vi "DrawFormattedMultilineString_SubVI.vi"(0 "PictureIn":picture, 1 "FormattedMultiLineStringIn":string="123<B>ABCD</B>456\nAAA<B>BBB<I>CCC<U>DDD</U>EEE</I>FFF</B>GGG\n<I>QWERTY</I>\n<U>D<B>123</B>D</U>E", 2 "TextRectangle":T2={"x"=10.0, "y"=10.0, "width"=150.0, "height"=200.0} {"height" format="%.2f"; "width" format="%.2f"; "y" format="%.2f"; "x" format="%.2f"}, 3 "Justification":T1=enum."RIGHT", 4 "GAP":i32, 5 "Font":T3={"Font Name:"="Arial", "Size"=14, "Strikeout?"=FALSE, "Italic?"=FALSE, "Underline?"=FALSE, "Outline?"=FALSE, "Shadow?"=FALSE, "Bold?"=FALSE}, 6 "scaleY":dbl=2.0, 7 "Color":u32(colorbox), 8 "scaleX":dbl=2.0) -> (14 "PictureOut":picture, 16 "NoChange":bool=TRUE)   [LabVIEW 2014, in "Graphics.lvclass"]
uses:
  <resource>/Framework/Providers/Open_GDS/UML/Graphics_class/Graphics.lvclass
  <resource>/Framework/Providers/Open_GDS/UML/General/Rectangle/Rectangle Rectangle2D.ctl
  <resource>/Framework/Providers/Open_GDS/UML/MultiLineString_class/JustificationType.ctl
  <resource>/Framework/Providers/Open_GDS/UML/MultiLineString_class/MultiLineString.lvclass
panel:
  # "Layout:\nRemove \\r\\n\nSplit in lines-array\nCalc width per char\nGet number of chars to use for line,\nif rest characters, add these to beggining of  lines-array.\nCalc Bound\nAdd \\r\\n where new lines breaks are"
  # "Drawing:\nRemove \\r, split line using \\n\nfor every line calc total length.\n\nFor each line\n  If left start\n  X=B.X+Gap\n  Right:\n  X=B.X+B.W-L.length-Gap\n  Center:\n  X=B.X+(B.W/2)-(L.length/2)\n  Draw Line\nEnd For"
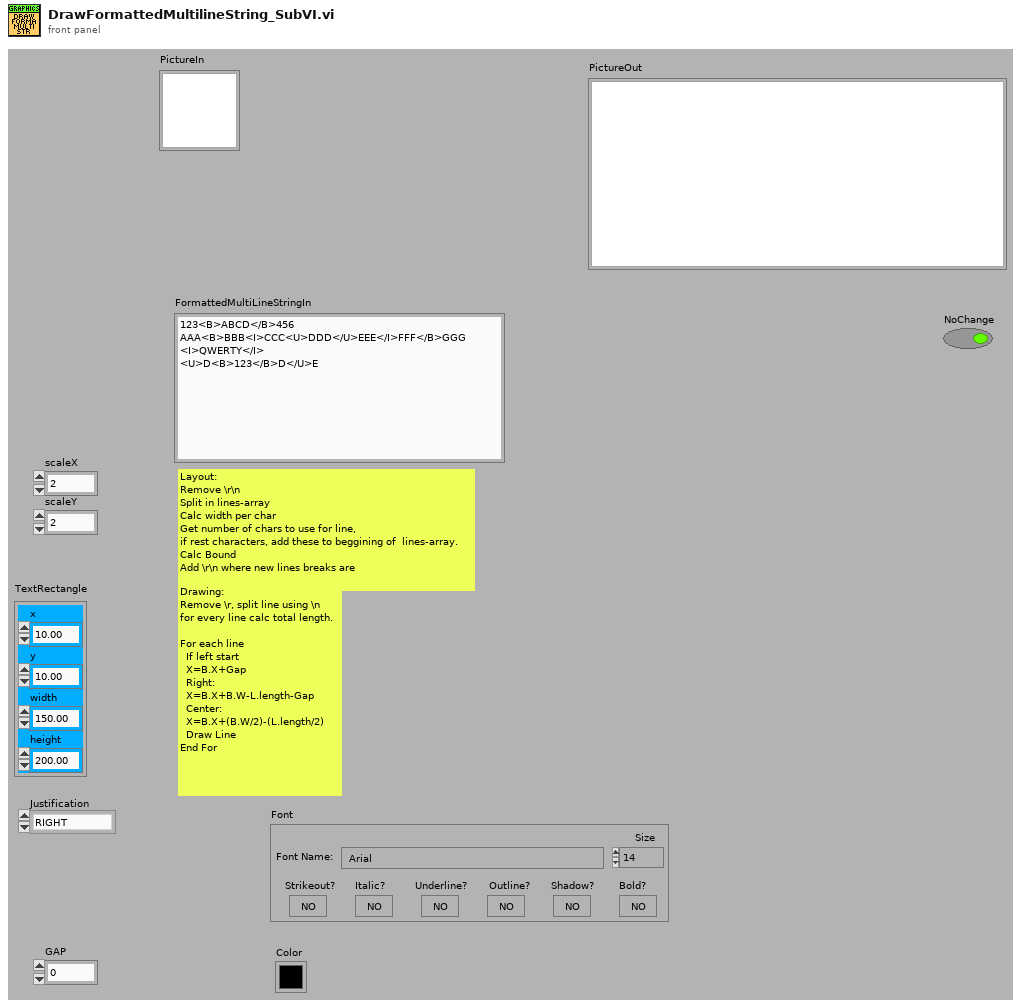
[diagram p1: front panel]
types:
  T1 = typedef "MultiLineString.lvclass/JustificationType.ctl" = enum16{"LEFT", "CENTER", "RIGHT"}
  T2 = typedef "Rectangle Rectangle2D.ctl" = cluster{"x":dbl, "y":dbl, "width":dbl, "height":dbl}
  T3 = cluster{"Font Name:":string, "Size":i16, "Strikeout?":bool, "Italic?":bool, "Underline?":bool, "Outline?":bool, "Shadow?":bool, "Bold?":bool}
  T4 = enum16{"User-specified Font", "Application Font", "System Font", "Dialog Font"}
  T5 = cluster{"horizontal":enum16{"left", "center", "right"}, "vertical":enum16{"top", "center", "bottom"}}
  T6 = cluster{cluster{"Start":i32, "Stop":i32, "Font":cluster{"Font Name:":string, "Size":i16, "Strikeout?":bool, "Italic?":bool, "Underline?":bool, "Outline?":bool, "Shadow?":bool, "Bold?":bool}, "Color":u32}[]}[]
  T7 = cluster{"Start":i32, "Stop":i32, "Font":cluster{"Font Name:":string, "Size":i16, "Strikeout?":bool, "Italic?":bool, "Underline?":bool, "Outline?":bool, "Shadow?":bool, "Bold?":bool}, "Color":u32}[]
  T8 = cluster{"left":i16, "top":i16, "right":i16, "bottom":i16}
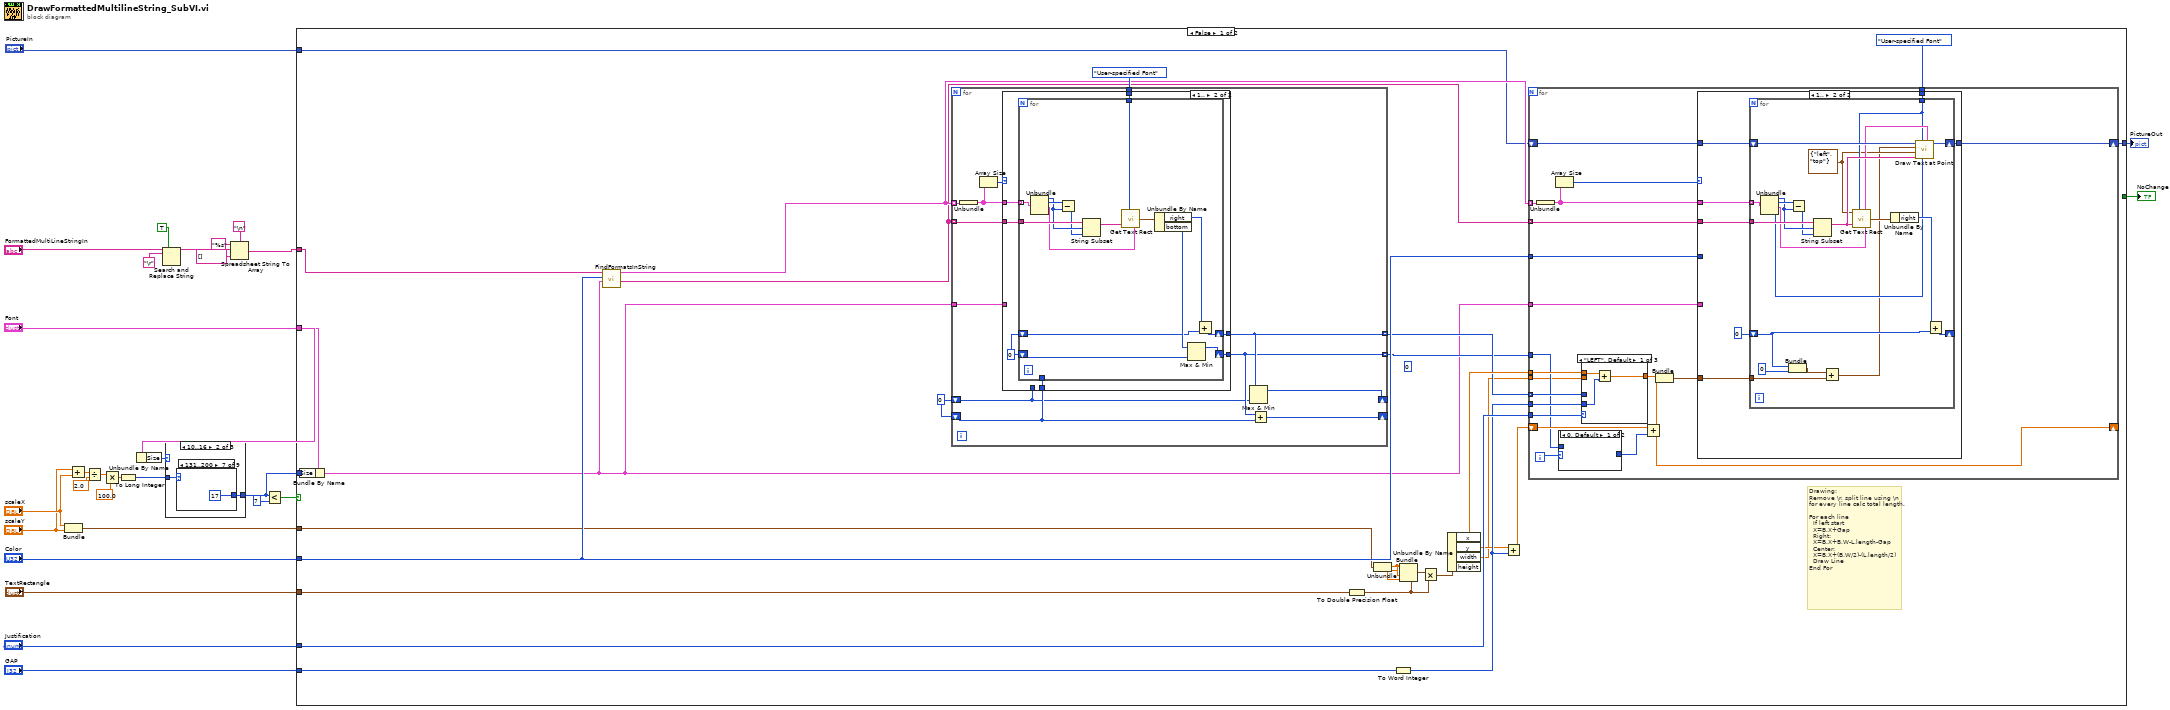
[diagram p0: block diagram]
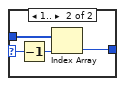
[diagram p2: hidden frame]
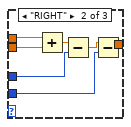
[diagram p3: hidden frame]
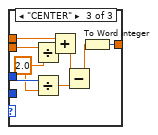
[diagram p4: hidden frame]
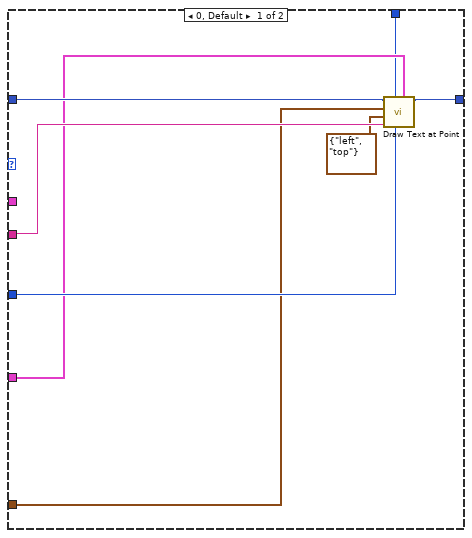
[diagram p5: hidden frame]
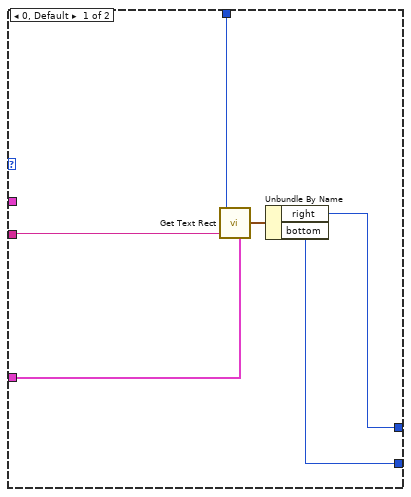
[diagram p6: hidden frame]
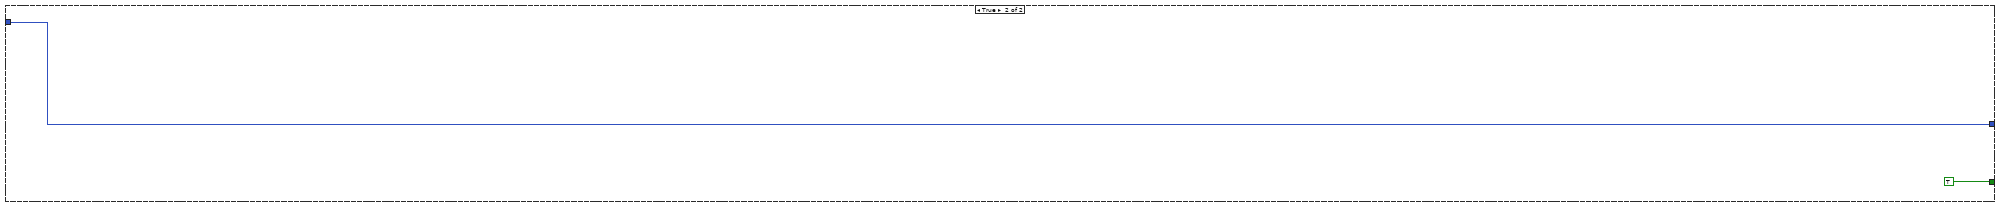
[diagram p7: hidden frame]
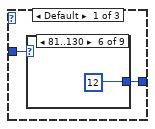
[diagram p8: hidden frame]
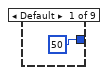
[diagram p9: hidden frame]
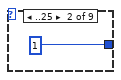
[diagram p10: hidden frame]
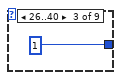
[diagram p11: hidden frame]
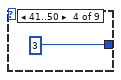
[diagram p12: hidden frame]
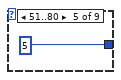
[diagram p13: hidden frame]
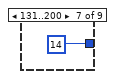
[diagram p14: hidden frame]
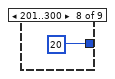
[diagram p15: hidden frame]
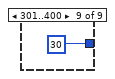
[diagram p16: hidden frame]
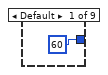
[diagram p17: hidden frame]
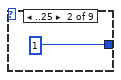
[diagram p18: hidden frame]
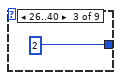
[diagram p19: hidden frame]
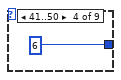
[diagram p20: hidden frame]
diagram:
  n1 = Bundle("scaleX"="scaleX", "scaleY"="scaleY") -> (w2:cluster{"scaleX":dbl, "scaleY":dbl})  [unwired: 1 out]
  n2 = Add(x="scaleY", y="scaleX") -> (x+y=w20:dbl)
  n3 = Divide(x=w20, y=2.0) -> (x/y=w18:dbl)
  n4 = Multiply(x=w18, y=100.0) -> (x*y=w16:dbl)
  n5 = To Long Integer(number=w16) -> (32bit integer=w15:i32)
  n6 = Unbundle By Name("Font") -> ("Size"=w10:i16)
  n7 = Search and Replace String(replace all?=TRUE ("replace all? (F)"), input string="FormattedMultiLineStringIn", search string="\r" ("delimiter (Tab)")) -> (result string=w23:string)  [unwired: 5 in, 3 out]
  n8 = case shown="10..16" w10 {
    tunnel: [w31 w42 w52] -> w9
    tunnel: w15 -> [w30 w41 w53]
    frame Default {
      n9 = case shown="81..130" w30 {
        tunnel: [i16 50 ("Size 9") i16 1 ("Size") i16 1 ("Size 2") i16 3 ("Size 3") i16 5 ("Size 4") i16 12 ("Size 5") i16 14 ("Size 6") i16 20 ("Size 7") i16 30 ("Size 8")] -> w31
        frame Default {
        }
        frame ..25 {
        }
        frame 26..40 {
        }
        frame 41..50 {
        }
        frame 51..80 {
        }
        frame 81..130 {
        }
        frame 131..200 {
        }
        frame 201..300 {
        }
        frame 301..400 {
        }
      }
    }
    frame 10..16 {
      n10 = case shown="131..200" w41 {
        tunnel: [i16 60 ("Size 9") i16 1 ("Size") i16 2 ("Size 2") i16 6 ("Size 3") i16 7 ("Size 4") i16 14 ("Size 5") i16 17 ("Size 6") i16 25 ("Size 7") i16 40 ("Size 8")] -> w42
        frame Default {
        }
        frame ..25 {
        }
        frame 26..40 {
        }
        frame 41..50 {
        }
        frame 51..80 {
        }
        frame 81..130 {
        }
        frame 131..200 {
        }
        frame 201..300 {
        }
        frame 301..400 {
        }
      }
    }
    frame 17.. {
      n11 = case shown="201..300" w53 {
        tunnel: [i16 82 ("Size") i16 2 ("Size") i16 5 ("Size") i16 7 ("Size") i16 12 ("Size") i16 18 ("Size") i16 26 ("Size") i16 36 ("Size") i16 55 ("Size")] -> w52
        frame Default {
        }
        frame ..25 {
        }
        frame 26..40 {
        }
        frame 41..50 {
        }
        frame 51..80 {
        }
        frame 81..130 {
        }
        frame 131..200 {
        }
        frame 201..300 {
        }
        frame 301..400 {
        }
      }
    }
  }
  n12 = Spreadsheet String To Array(delimiter (Tab)="\n", format string="%s", spreadsheet string=w23, array type (2D Dbl)=string[] []) -> (array=w27:string[])
  n13 = Less?(x=w9, y=i16 7) -> (x < y?=w4:bool)
  n14 = case shown="False" w4 {
    tunnel: w27 -> [w90 _]
    tunnel: [w85 w211] -> w22
    tunnel: "TextRectangle" -> [w84 _]
    tunnel: "Color" -> [w83 _]
    tunnel: w9 -> [w82 _]
    tunnel: "Justification" -> [w80 _]
    tunnel: "GAP" -> [w79 _]
    tunnel: "Font" -> [w71 _]
    tunnel: w2 -> [w69 _]
    tunnel: "PictureIn" -> [w64 w211]
    tunnel: [_ TRUE] -> w3
    frame False {
      (unwired) 0 ("index")
      w88 = i16 0
      # "Drawing:\nRemove \\r, split line using \\n\nfor every line calc total length.\n\nFor each line\n  If left start\n  X=B.X+Gap\n  Right:\n  X=B.X+B.W-L.length-Gap\n  Center:\n  X=B.X+(B.W/2)-(L.length/2)\n  Draw Line\nEnd For"
      n15 = Bundle By Name(cluster=w71, "Size"=w82) -> (w63:T3)
      n16 = call <resource>:"FindFormatsInString.vi"("Font"=w63, "Color"=w83, "StringsIn"=w90) -> ("StringsOut"=w86:string[], "Formats"=w87:T6)  [unwired: 7 in]
      n17 = for {
        tunnel: w87 -> [w181] mode=indexing
        tunnel: w86 -> [w180] mode=indexing
        tunnel: T4."User-specified Font" ("desired font(Application)") -> [w179]
        shift-right: [w178] -> _
        shift-left: w88 -> [w171]
        shift-right: [w177] -> _
        shift-left: w88 -> [w170]
        tunnel: [w176] -> w78 mode=indexing
        tunnel: [w175] -> w73 mode=indexing
        tunnel: w63 -> [w172]
        n18 = Unbundle(w181) -> (w174:T7)
        n19 = Array Size(array=w174) -> (size(s)=w173:i32)
        n20 = case shown="1.." w173 {
          tunnel: w180 -> [w183 w194]
          tunnel: w179 -> [w184 w193]
          tunnel: [w185 w191] -> w176
          tunnel: [w186 w190] -> w175
          tunnel: w174 -> [_ w189]
          tunnel: w172 -> [w182 _]
          tunnel: w171 -> [_ w188]
          tunnel: w170 -> [_ _]
          frame 0, Default {
            n21 = call <vilib>:"Get Text Rect.vi"("desired font(Application)"=w184, "text"=w183, "[user-specified font]"=w182) -> ("rect"=w187:T8)  [unwired: 6 in]
            n22 = Unbundle By Name(w187) -> ("right"=w185:i16, "bottom"=w186:i16)
          }
          frame 1.. {
            w192 = i16 0
            n23 = for {
              tunnel: w194 -> [w208]
              tunnel: w189 -> [w209] mode=indexing
              tunnel: w193 -> [w196]
              shift-right: [w199] -> w191
              shift-left: w192 -> [w197]
              shift-right: [w201] -> w190
              shift-left: w192 -> [w202]
              tunnel: w188 -> [_]
              n24 = Unbundle(w209) -> ("Start"=w206:i32, "Stop"=w207:i32, "Font"=w195:T3)  [unwired: 1 out]
              n25 = Subtract(x=w207, y=w206) -> (x-y=w205:i32)
              n26 = String Subset(string=w208, offset (0)=w206, length (rest)=w205) -> (substring=w198:string)
              n27 = call <vilib>:"Get Text Rect.vi"("desired font(Application)"=w196, "text"=w198, "[user-specified font]"=w195) -> ("rect"=w204:T8)  [unwired: 6 in]
              n28 = Unbundle By Name(w204) -> ("right"=w200:i16, "bottom"=w203:i16)
              n29 = Max & Min(x=w203, y=w202) -> (max(x,y)=w201:i16)  [unwired: 1 out]
              n30 = Add(x=w200, y=w197) -> (x+y=w199:i16)
            }
          }
        }
        n31 = Max & Min(x=w176, y=w170) -> (max(x,y)=w177:i16)  [unwired: 1 out]
        n32 = Add(x=w175, y=w171) -> (x+y=w178:i16)
      }
      n33 = To Double Precision Float(number=w84) -> (double precision float=w66:T2)
      n34 = Unbundle(w69) -> ("scaleX"=w68:dbl, "scaleY"=w67:dbl)
      n35 = To Word Integer(number=w79) -> (16bit integer=w77:i16)
      n36 = Bundle(cluster=w66, "x"=w68, "y"=w67, "width"=w68, "height"=w67) -> (w65:T2)
      n37 = Multiply(x=w65, y=w66) -> (x*y=w70:T2)
      n38 = Unbundle By Name(w70) -> ("x"=w81:dbl, "y"=w76:dbl, "width"=w72:dbl)  [unwired: 1 out]
      n39 = Add(x=w76, y=w77) -> (x+y=w75:dbl)
      n40 = for {
        tunnel: w87 -> [w111] mode=indexing
        tunnel: w86 -> [w110] mode=indexing
        tunnel: w63 -> [w107]
        shift-right: [w105] -> w85
        shift-left: w64 -> [w106]
        tunnel: w83 -> [w104]
        tunnel: w81 -> [w98]
        tunnel: w80 -> [w99]
        tunnel: w77 -> [w101]
        tunnel: w78 -> [w100] mode=indexing
        tunnel: w73 -> [w94]
        shift-right: [w96] -> _
        shift-left: w75 -> [w102]
        tunnel: T4."User-specified Font" ("desired font(Application)") -> [w95]
        tunnel: w72 -> [w91]
        i -> [w92]
        n41 = Unbundle(w111) -> (w109:T7)
        n42 = Array Size(array=w109) -> (size(s)=w108:i32)
        n43 = case shown="0, Default" w92 {
          selector: w92 -> [_ w112]
          tunnel: w94 -> [_ w115]
          tunnel: [_ w113] -> w93
          frame 0, Default {
          }
          frame 1.. {
            n44 = Decrement(x=w112) -> (x-1=w114:i32)
            n45 = Index Array(array=w115, index=w114) -> (element=w113:i16)
          }
        }
        n46 = case shown="\"LEFT\", Default" w99 {
          tunnel: w100 -> [_ w121 w128]
          tunnel: w98 -> [w118 w119 w133]
          tunnel: w101 -> [w117 w125 _]
          tunnel: [w116 w124 w132] -> w103
          tunnel: w91 -> [_ w120 w131]
          frame "LEFT", Default {
            n47 = Add(x=w118, y=w117) -> (x+y=w116:dbl)
          }
          frame "RIGHT" {
            n48 = Add(x=w119, y=w120) -> (x+y=w123:dbl)
            n49 = Subtract(x=w123, y=w121) -> (x-y=w122:dbl)
            n50 = Subtract(x=w122, y=w125) -> (x-y=w124:dbl)
          }
          frame "CENTER" {
            w127 = 2.0 ("y")
            n51 = Divide(x=w131, y=w127) -> (x/y=w134:dbl)
            n52 = Divide(x=w128, y=w127) -> (x/y=w126:dbl)
            n53 = Add(x=w133, y=w134) -> (x+y=w130:dbl)
            n54 = Subtract(x=w130, y=w126) -> (x-y=w129:dbl)
            n55 = To Word Integer(number=w129) -> (16bit integer=w132:i16)
          }
        }
        n56 = Add(x=w102, y=w93) -> (x+y=w96:dbl)
        n57 = Bundle(w103, w96) -> (w97:cluster{dbl, dbl})  [unwired: 1 in]
        n58 = case shown="1.." w108 {
          tunnel: w110 -> [w140 w149]
          tunnel: w109 -> [_ w147]
          tunnel: w107 -> [w137 _]
          tunnel: w106 -> [w142 w146]
          tunnel: [w141 w145] -> w105
          tunnel: w104 -> [w138 _]
          tunnel: w97 -> [w135 w143]
          tunnel: w95 -> [w136 w144]
          frame 0, Default {
            n59 = call <vilib>:"Draw Text at Point.vi"("[user-specified font]"=w137, "text color(black)"=w138, "desired font(Application)"=w136, "text"=w140, "alignment(left, top)"=T5 {"horizontal"=enum."left", "vertical"=enum."top"}, "origin"=w135, "picture"=w142) -> ("new picture"=w141:picture)  [unwired: 3 in, 1 out]
          }
          frame 1.. {
            n60 = for {
              tunnel: w149 -> [w168]
              tunnel: w147 -> [w169] mode=indexing
              shift-right: [w162] -> _
              shift-left: i16 0 -> [w158]
              shift-right: [w160] -> w145
              shift-left: w146 -> [w161]
              tunnel: w143 -> [w155]
              tunnel: w144 -> [w152]
              w151 = T5 {"horizontal"=enum."left", "vertical"=enum."top"} ("alignment(left, top)")
              n61 = Unbundle(w169) -> ("Start"=w166:i32, "Stop"=w167:i32, "Font"=w156:T3, "Color"=w157:u32)
              n62 = Bundle(w158, i16 0) -> (w154:cluster{i16, i16})  [unwired: 1 in]
              n63 = Subtract(x=w167, y=w166) -> (x-y=w165:i32)
              n64 = String Subset(string=w168, offset (0)=w166, length (rest)=w165) -> (substring=w159:string)
              n65 = Add(x=w154, y=w155) -> (x+y=w150:cluster{dbl, dbl})
              n66 = call <vilib>:"Get Text Rect.vi"("alignment(left, top)"=w151, "desired font(Application)"=w152, "text"=w159, "[user-specified font]"=w156) -> ("rect"=w164:T8)  [unwired: 5 in]
              n67 = Unbundle By Name(w164) -> ("right"=w163:i16)
              n68 = call <vilib>:"Draw Text at Point.vi"("[user-specified font]"=w156, "text color(black)"=w157, "desired font(Application)"=w152, "text"=w159, "alignment(left, top)"=w151, "origin"=w150, "picture"=w161) -> ("new picture"=w160:picture)  [unwired: 3 in, 1 out]
              n69 = Add(x=w163, y=w158) -> (x+y=w162:i16)
            }
          }
        }
      }
    }
    frame True {
    }
  }
  "PictureOut" <- w22
  "NoChange" <- w3
